vi "Read State from File.vi"(0 "Display State In":T2, 5 "tdms file":refnum<k34>, 7 "Lable.Text":string, 9 "Container State":T3, 11 "error in (no error)":errorcluster) -> (4 "Display State Out":T2, 6 "tdms file out":refnum<k34>, 15 "error out":errorcluster)   [LabVIEW 2015, in "Dynamic Device List.xctl"]
uses:
  Dynamic Device List.xctl
  <vilib>/_xctls/Container State.ctl
  Dynamic FP container.llb/Dynamic FP State.ctl
  Device/Device.lvclass
  Device List State.ctl
  Dynamic FP XControl/Name type and data.ctl
  Device/Device type.ctl
  <vilib>/_xctls/XControlSupport.lvlib
panel:
  in  "Device List State":T1
  out "Device List State out":T1
  # "Add Controls & Indicators that form the parameters of the method here. Hook them to the connector pane. Do not delete the controls & indicators that are already hooked to the connector pane.\n \nTo setup the parameters  for this method, right click on this item in the Project Tree & select \"Configure Method...\"."
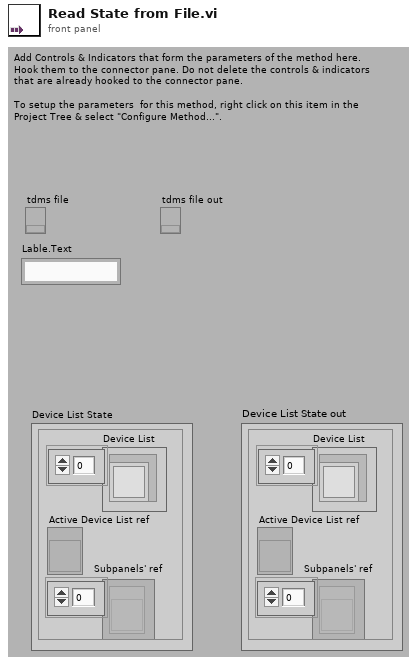
[diagram p1: front panel]
types:
  T1 = typedef "Device List State.ctl" = cluster{"Device List":refnum<class "Device.lvclass">[], "Active Device List ref":refnum<vi>, "Subpanels' ref":refnum<vi>[]}
  T2 = typedef "Dynamic Device List.xctl/Dynamic FP State.ctl" = cluster{"Complete device list":refnum<class "Device.lvclass">[], "Boolean test":bool, "Selected devices":u16[]}
  T3 = typedef "XControlSupport.lvlib/Container State.ctl" = cluster{"Indicator?":bool, "Run Mode?":bool, " Refnum":refnum<vi>}
  T4 = typedef "Name type and data.ctl" = cluster{"Front Panel Data":variant, "Device type":T5, "Name":string}
  T5 = typedef "Device type.ctl" = enum16{"NONE", "Neocera 21", "LakeShore 335", "LakeShore 340", "LkShr 340 chA&B", "LakeShore 370", "SRS 850", "SRS 830", "LR 700", "EG&G 5302", "EG&G 7260", "EG&G 7280", "AH 2500", "Keithley meter", "Keithley electrometer", "Keithley 182", "HP 5385", "HP 53181", "HP 53132", "ITC503", "IPS120", "Oxford Mercury IPS", "Oxford PS", "Test", "DC Facility Magnet", "Cryomagnetics PS", "Keithley 2400", "Keithley current source", "Cryo-Con 22C", "HP87NN", "HP4395A"}
  T6 = cluster{"Saved device":i32, "Present device":i32}[]
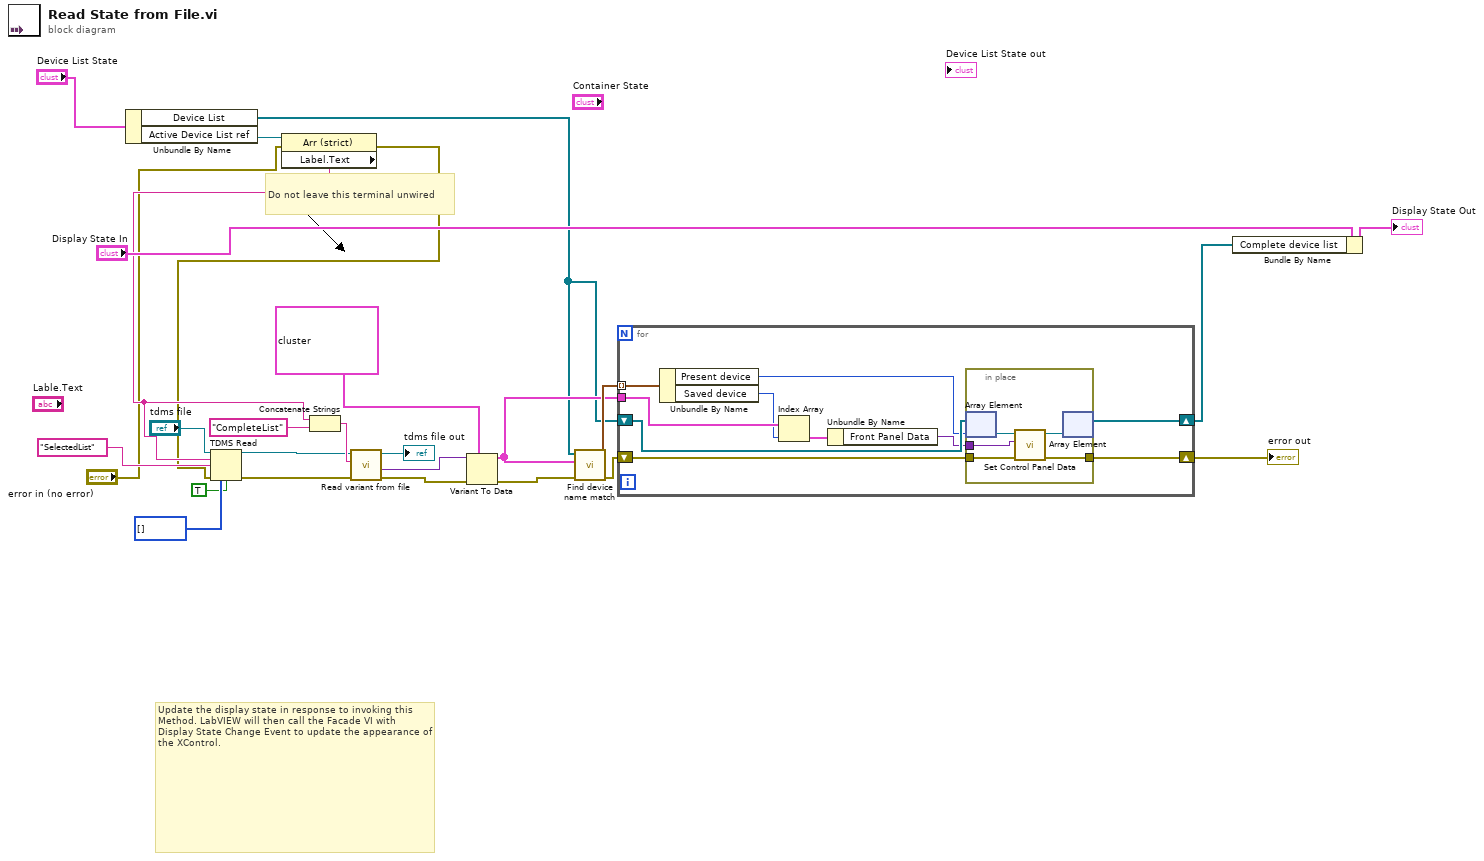
[diagram p0: block diagram]
diagram:
  # "Do not leave this terminal unwired"
  # "Update the display state in response to invoking this Method. LabVIEW will then call the Facade VI with Display State Change Event to update the appearance of the XControl."
  n1 = Unbundle By Name("Device List State") -> ("Device List"=w5:refnum<class "Device.lvclass">[], "Active Device List ref"=w4:refnum<vi>)
  n2 = property class="Arr (strict)"(reference=w4, error in="error in (no error)") -> (error out=w1:errorcluster, "Label.Text"=w3:string)  [unwired: 1 out]
  n3 = TDMS Read(0:"tdms file", 5:w3, 7:"SelectedList" ("string"), 11:w1, 12:u16[] [] ("Selected devices"), 13:TRUE ("return channels in file order? (F)")) -> (4:w22:refnum<k34>, 15:w23:errorcluster)  [unwired: 2 in, 4 out]
  n4 = Concatenate Strings(w3, "CompleteList" ("string")) -> (w24:string)
  n5 = call "Read variant from file.vi"("error in (no error)"=w23, "group name in"=w24, "tdms file"=w22) -> ("error out"=w17:errorcluster, "variant out"=w19:variant, "tdms file out"=→"tdms file out":refnum<k34>)  [unwired: 6 in]
  n6 = Variant To Data(error in=w17, type=T4[] [{"Front Panel Data"=variant, "Device type"=enum."NONE", "Name"=""}], Variant=w19) -> (data=w12:T4[], error out=w14:errorcluster)
  n7 = call "Find device name match.vi"("error in"=w14, "Saved names and data"=w12, "Device list"=w5) -> ("error out"=w11:errorcluster, "Matching pairs"=w13:T6)  [unwired: 7 in]
  n8 = for {
    tunnel: w13 -> [w35] mode=indexing
    shift-right: [w31] -> w9
    shift-left: w5 -> [w36]
    tunnel: w12 -> [w33]
    shift-right: [w28] -> w8
    shift-left: w11 -> [w29]
    n9 = Unbundle By Name(w35) -> ("Present device"=w34:i32, "Saved device"=w32:i32)
    n10 = Index Array(array=w33, index=w32) -> (element=w30:T4)
    n11 = Unbundle By Name(w30) -> ("Front Panel Data"=w27:variant)
    n12 = in-place {
      in-place-border: w27 -> [w39]
      in-place-border: w29 -> [w38]
      in-place-border: [w37] -> w28
      n13 = in-place-array #1(w36, w34) -> (w41:refnum<class "Device.lvclass">)
      n14 = call "Set Control Panel Data.vi"("error in (no error)"=w38, "Data"=w39, "Device in"=w41) -> ("error out"=w37:errorcluster, "Device out"=w40:refnum<class "Device.lvclass">)  [unwired: 7 in]
      n15 = in-place-array #1(w40) -> (w31:refnum<class "Device.lvclass">[])  [unwired: 1 out]
    }
  }
  "error out" <- w8
  n16 = Bundle By Name(cluster="Display State In", "Complete device list"=w9) -> (→"Display State Out":T2)
